vi "construct tag.vi"(8 "raw default":variant, 9 "metadata":string, 10 "data type":T1, 11 "name":string) -> (3 "system tag out":refnum<class "data bus tag description.lvclass">)   [LabVIEW 2013, in "data bus tag description.lvclass"]
doc: "Creates a new instance of the tag descriptor class."
uses:
  data bus tag description.lvclass
  Data Type.ctl
  data bus tag description.lvclass/data bus tag description.ctl
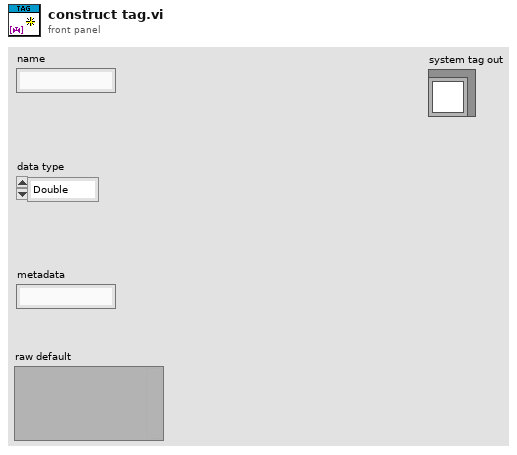
[diagram p1: front panel]
types:
  T1 = typedef "data bus tag description.lvclass/Data Type.ctl" = enum16{"Double", "I64", "Boolean", "Array of Double", "Array of I64", "Variant"}
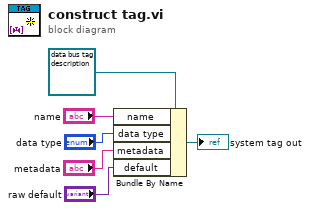
[diagram p0: block diagram]
diagram:
  n1 = Bundle By Name(cluster=refnum<class "data bus tag description.lvclass"> refnum ("system tag in"), "name"="name", "data type"="data type", "metadata"="metadata", "default"="raw default") -> (→"system tag out":refnum<class "data bus tag description.lvclass">)
